vi "Module Timeout--constant.vi"() -> (3 "Module Timeout":i32)   [LabVIEW 2023, in "Dispatcher.lvlib"]
doc: "A module-wide common value to use as the timeout for various synchronization actions.\n_____\nBased on DQMH Project Template 6.1.0.94."
uses:
  Dispatcher.lvlib
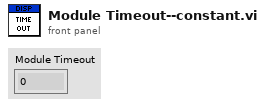
[diagram p1: front panel]
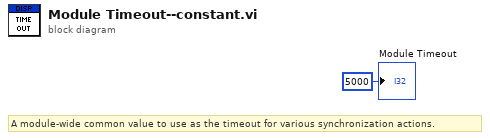
[diagram p0: block diagram]
diagram:
  # "A module-wide common value to use as the timeout for various synchronization actions."
  "Module Timeout" <- 5000 ("Module Timeout")
